vi "reflectionPool__ogtk.vi"(8 "error in (no error)":errorcluster, 9 "objectToAddToPool":refnum<class>, 10 "action":T1) -> (0 "error out":errorcluster, 1 "allClassNames":string[](array[string]), 2 "entireHierarchy":string[][](array[string]), 3 "classHierarchyLUT":variant, 4 "classPrivateDataLUT":variant, 6 "classVersionNumbersLUT":variant)   [LabVIEW 2023, in "openg_variant.lvlib" / "Reflection__ogtk.lvclass"]
doc: "GCraftsman JSON Object Serialization Toolkit\nwww.GCraftsman.com\nCopyright (c) 2017, GCraftsman"
uses:
  Reflection__ogtk.lvclass
  ClassLoader__ogtk.lvclass
  reflectionPoolAction__ogtk.ctl
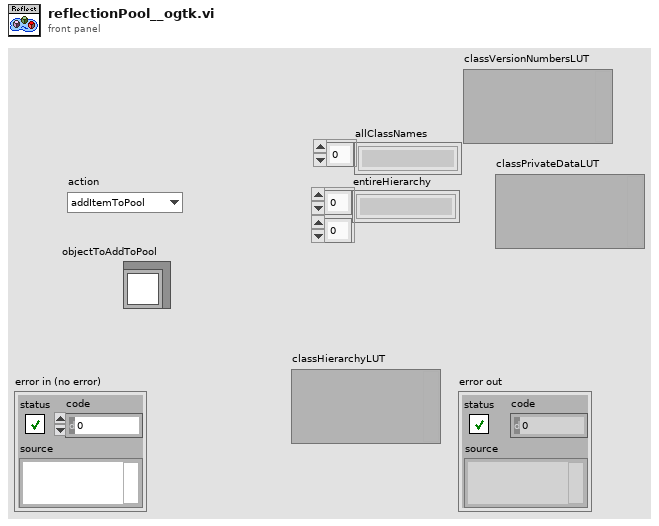
[diagram p1: front panel]
types:
  T1 = typedef "openg_variant.lvlib/Reflection__ogtk.lvclass/reflectionPoolAction__ogtk.ctl" = enum16{"addItemToPool", "getAncestry"}
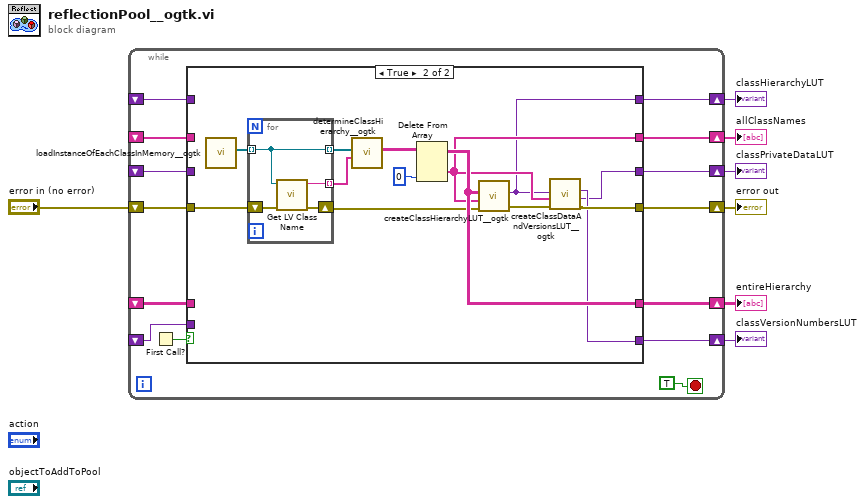
[diagram p0: block diagram]
diagram:
  n1 = while {
    shift-right: [w18] -> w6
    shift-left: _ -> [w20]
    shift-right: [w17] -> w7
    shift-left: _ -> [w16]
    shift-right: [w14] -> w4
    shift-left: "error in (no error)" -> [w15]
    shift-right: [w13] -> w3
    shift-left: _ -> [w12]
    shift-right: [w11] -> w2
    shift-left: _ -> [w10]
    shift-right: [w9] -> w1
    shift-left: _ -> [w8]
    stop <- TRUE stop-if-true
    n2 = First Call?() -> (First Call?: T/F=w21:bool)
    n3 = case shown="True" w21 {
      tunnel: w20 -> [w27 _]
      tunnel: [w27 w35] -> w18
      tunnel: [w26 w33] -> w17
      tunnel: w16 -> [w26 _]
      tunnel: w10 -> [w23 _]
      tunnel: w15 -> [w25 w36]
      tunnel: [w25 w30] -> w14
      tunnel: [w24 w31] -> w13
      tunnel: w12 -> [w24 _]
      tunnel: [w23 w29] -> w11
      tunnel: [w22 w28] -> w9
      tunnel: w8 -> [w22 _]
      frame False {
      }
      frame True {
        n4 = call "loadInstanceOfEachClassInMemory__ogtk.vi"() -> ("AllClassesInMemory"=w41:refnum<class>[])  [unwired: 11 in]
        n5 = for {
          tunnel: w41 -> [w45] mode=indexing
          tunnel: [w44] -> w39 mode=indexing
          tunnel: [w45] -> w40 mode=indexing
          shift-right: [w42] -> w34
          shift-left: w36 -> [w43]
          n6 = call <vilib>:"Get LV Class Name.vi"("error in (no error)"=w43, "object"=w45) -> ("error out"=w42:errorcluster, "class name"=w44:string)  [unwired: 8 in]
        }
        n7 = call "determineClassHierarchy__ogtk.vi"("classNames"=w39, "classObjects"=w40) -> ("hierarchy"=w37:string[][])  [unwired: 8 in, 1 out]
        n8 = Delete From Array(array=w37, index (col)=0 ("disabled index (col)")) -> (deleted portion=w33:string[], array with subset deleted=w35:string[][])  [unwired: 2 in]
        n9 = call "createClassHierarchyLUT__ogtk.vi"("error in (no error)"=w34, "allClassNames"=w33, "entireHierarchy"=w35) -> ("error out"=w32:errorcluster, "classHierarchyLUT"=w31:variant)  [unwired: 7 in]
        n10 = call "createClassDataAndVersionsLUT__ogtk.vi"("error in (no error)"=w32, "allClassNames"=w33, "classHierarchyLUT"=w31) -> ("error out"=w30:errorcluster, "classPrivateDataLUT"=w28:variant, "classVersionNumbersLUT"=w29:variant)  [unwired: 5 in, 1 out]
      }
    }
  }
  "error out" <- w4
  "allClassNames" <- w7
  "entireHierarchy" <- w6
  "classHierarchyLUT" <- w3
  "classVersionNumbersLUT" <- w2
  "classPrivateDataLUT" <- w1
